vi "DQMH_Name Module.vi"(8 "error in":errorcluster, 10 "String":string, 11 "Module ID in":i32) -> (0 "error out":errorcluster, 3 "input cluster":T1)   [LabVIEW 2025]
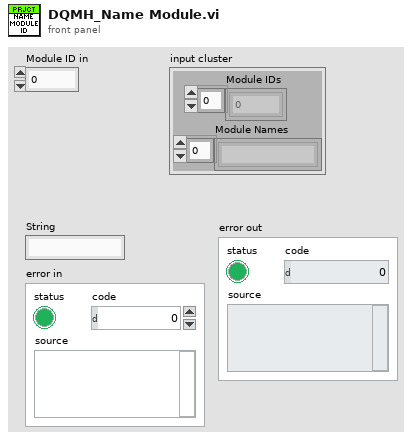
[diagram p1: front panel]
types:
  T1 = cluster{"Module IDs":i32[], "Module Names":string[]}
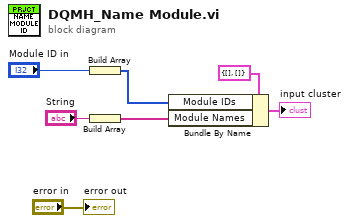
[diagram p0: block diagram]
diagram:
  n1 = Build Array("Module ID in") -> (w4:i32[])
  n2 = Build Array("String") -> (w5:string[])
  n3 = Bundle By Name(cluster=T1 {"Module IDs"=[], "Module Names"=[]} ("input cluster"), "Module IDs"=w4, "Module Names"=w5) -> (→"input cluster":T1)
  "error out" <- "error in"
